vi "LVPortDeleteTempValue.vi"(10 "Object ID":i32, 11 "pID":string) -> (3 "Found and Removed":bool)   [LabVIEW 2017]
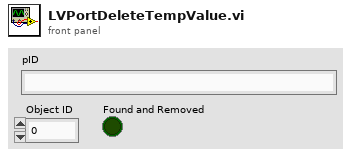
[diagram p1: front panel]
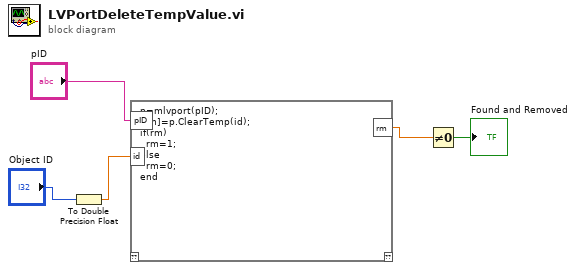
[diagram p0: block diagram]
diagram:
  n1 = To Double Precision Float(number="Object ID") -> (double precision float=w4:dbl)
  n2 = script code="p=mlvport(pID);\n[rm]=p.ClearTemp(id);\nif(rm)\n  rm=1;\nelse\n  rm=0;\nend"("pID"="pID", "id"=w4) -> ("rm"=w2:dbl)  [unwired: 1 in, 1 out]
  n3 = Not Equal To 0?(x=w2) -> (x != 0?=→"Found and Removed":bool)
